vi "testDigitalOutputs.vi"(8 "error in (no error)":errorcluster, 9 "Digital Output Values":T1, 10 "Digital Output Value":i32=-1 min=-1 max=16383, 11 "ILC in":refnum<class "ILC.lvclass">) -> (0 "error out":errorcluster, 3 "ILC out":refnum<class "ILC.lvclass">)   [LabVIEW 2015, in "ILCCommon.lvlib" / "ILC.lvclass"]
uses:
  <userlib>/Common/ILC/ILC/ILC.lvclass
  <userlib>/Common/ILC/Typedefs/DigitalOutputValues.ctl
  <userlib>/Common/ILC/ILC/ILC.lvclass/ILC.ctl
  <userlib>/Common/SerialProtocols/SerialCommunicator/SerialCommunicator.lvclass
  <userlib>/Common/ILC/Typedefs/ILCTypedefs.lvlib
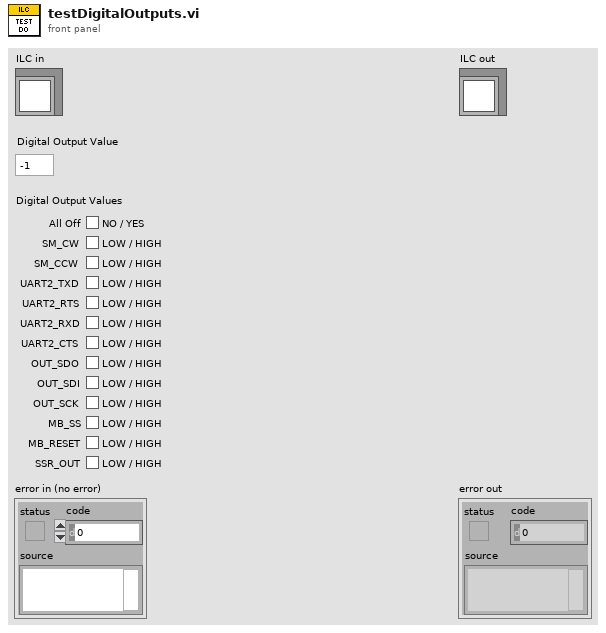
[diagram p1: front panel]
types:
  T1 = typedef "ILCCommon.lvlib/ILCTypedefs.lvlib/DigitalOutputValues.ctl" = cluster{"All Off":bool, "SM_CW":bool, "SM_CCW":bool, "UART2_TXD":bool, "UART2_RTS":bool, "UART2_RXD":bool, "UART2_CTS":bool, "OUT_SDO":bool, "OUT_SDI":bool, "OUT_SCK":bool, "MB_SS":bool, "MB_RESET":bool, "SSR_OUT":bool}
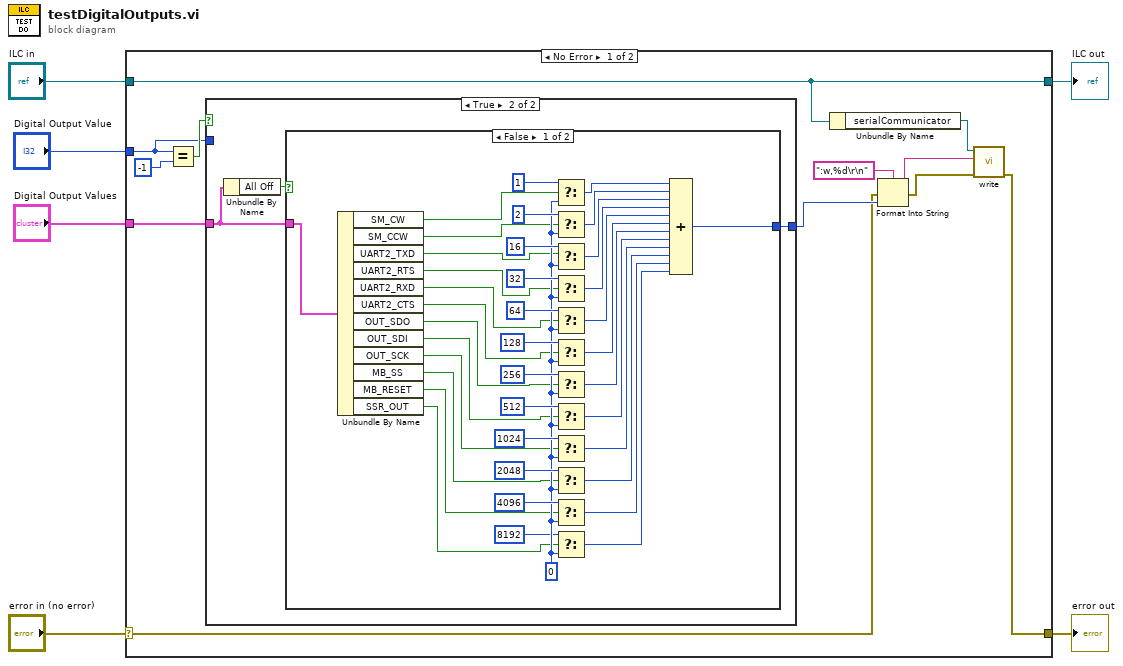
[diagram p0: block diagram]
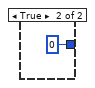
[diagram p3: hidden frame]
diagram:
  n1 = case shown="No Error" "error in (no error)" {
    selector: "error in (no error)" -> [w10 w64]
    tunnel: [w7 w64] -> w5
    tunnel: [w14 w63] -> w3
    tunnel: "ILC in" -> [w14 w63]
    tunnel: "Digital Output Value" -> [w15 _]
    tunnel: "Digital Output Values" -> [w16 _]
    frame No Error {
      n2 = Equal?(x=w15, y=-1) -> (x = y?=w18:bool)
      n3 = case shown="True" w18 {
        tunnel: w16 -> [_ w20]
        tunnel: w15 -> [w19 _]
        tunnel: [w19 w21] -> w12
        frame False {
        }
        frame True {
          n4 = Unbundle By Name(w20) -> ("All Off"=w22:bool)
          n5 = case shown="False" w22 {
            tunnel: [w61 0] -> w21
            tunnel: w20 -> [w35 _]
            frame False {
              w38 = 0
              n6 = Unbundle By Name(w35) -> ("SM_CW"=w34:bool, "SM_CCW"=w33:bool, "UART2_TXD"=w32:bool, "UART2_RTS"=w31:bool, "UART2_RXD"=w30:bool, "UART2_CTS"=w29:bool, "OUT_SDO"=w28:bool, "OUT_SDI"=w27:bool, "OUT_SCK"=w26:bool, "MB_SS"=w25:bool, "MB_RESET"=w24:bool, "SSR_OUT"=w23:bool)
              n7 = Select(t=1, s=w34, f=w38) -> (s? t:f=w60:i32)
              n8 = Select(t=2, s=w33, f=w38) -> (s? t:f=w58:i32)
              n9 = Select(t=16, s=w32, f=w38) -> (s? t:f=w56:i32)
              n10 = Select(t=32, s=w31, f=w38) -> (s? t:f=w54:i32)
              n11 = Select(t=64, s=w30, f=w38) -> (s? t:f=w52:i32)
              n12 = Select(t=128, s=w29, f=w38) -> (s? t:f=w50:i32)
              n13 = Select(t=256, s=w28, f=w38) -> (s? t:f=w48:i32)
              n14 = Select(t=512, s=w27, f=w38) -> (s? t:f=w46:i32)
              n15 = Select(t=1024, s=w26, f=w38) -> (s? t:f=w43:i32)
              n16 = Select(t=2048, s=w25, f=w38) -> (s? t:f=w42:i32)
              n17 = Select(t=4096, s=w24, f=w38) -> (s? t:f=w40:i32)
              n18 = Select(t=8192, s=w23, f=w38) -> (s? t:f=w37:i32)
              n19 = Compound Arithmetic op=ADD(w60, w58, w56, w54, w52, w50, w48, w46, w43, w42, w40, w37) -> (w61:i32)
            }
            frame True {
            }
          }
        }
      }
      n20 = Unbundle By Name(w14) -> ("serialCommunicator"=w13:refnum<class "SerialCommunicator.lvclass">)
      n21 = Format Into String(format string=":w,%d\r\n", error in=w10, w12) -> (resulting string=w8:string, error out=w9:errorcluster)  [unwired: 1 in]
      n22 = call-dynamic "write.vi"("error in (no error)"=w9, "writeString"=w8, "SerialCommunicator in"=w13) -> ("error out"=w7:errorcluster)  [unwired: 7 in, 1 out]
    }
    frame Error {
    }
  }
  "error out" <- w5
  "ILC out" <- w3
